vi "convert.vi"() -> ()   [LabVIEW 2013]
uses:
  errors/severity.ctl
  <vilib>/addons/JSON API/Variant JSON/Variant to JSON.vi
  <vilib>/addons/JSON API/JSON Value/Get as JSON string (pretty).vi
  errors/exception.lvlib
  <vilib>/addons/JSON API/Get Polymorphic/JSON GetSet.lvlib
  <vilib>/addons/JSON API/Variant JSON/Variant JSON.lvlib
  <vilib>/addons/JSON API/JSON Value/JSON Value.lvclass
panel:
  out "LabVIEW Text":string
  out "error in":errorcluster
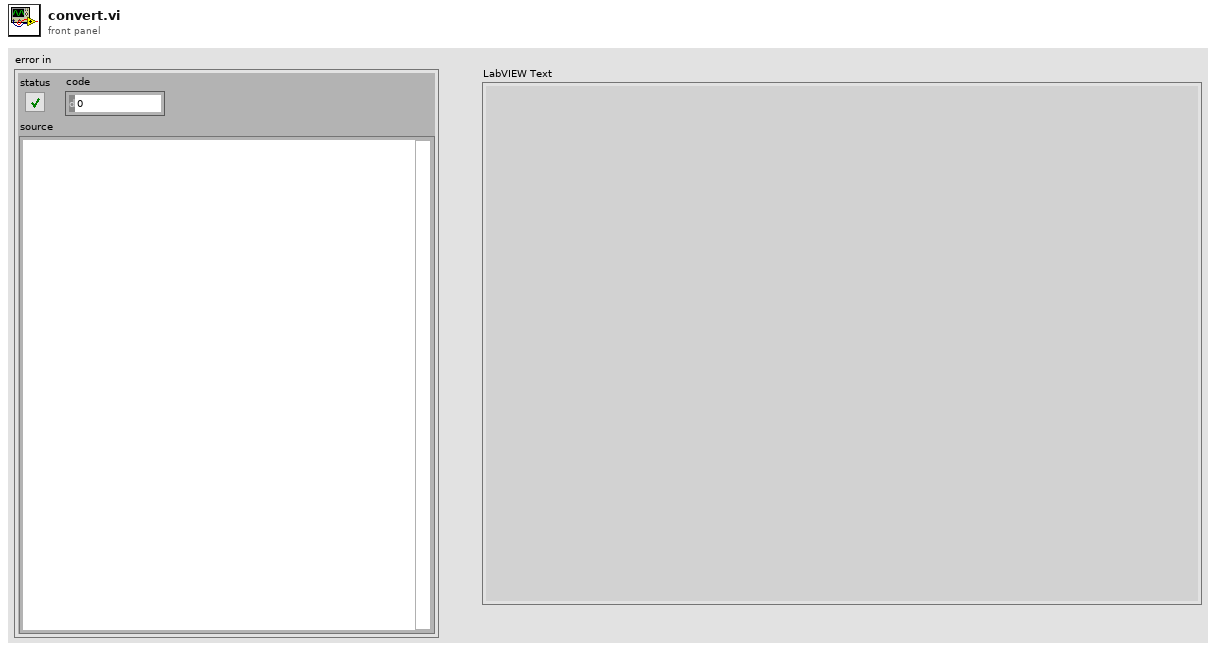
[diagram p1: front panel]
types:
  T1 = typedef "exception.lvlib/severity.ctl" = enum8{"unspecified", "operation failed", "data corruption", "system corruption", "critical unknown state"}
  T2 = typedef "exception.lvlib/exception.ctl" = cluster{"code":i32, "context":T3, "properties":variant}
  T3 = typedef "exception.lvlib/context.ctl" = enum16{"developer", "user interface", "standard", "limited", "deterministic"}
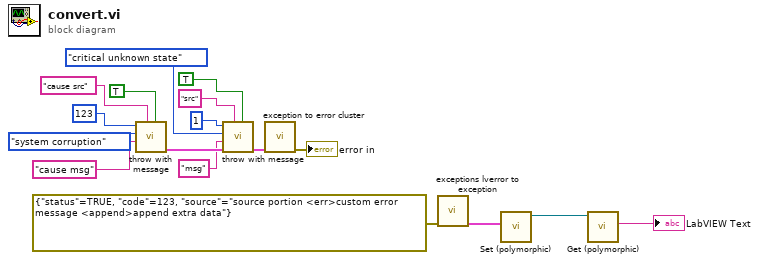
[diagram p0: block diagram]
diagram:
  n1 = call "throw with message.vi"("call chain?"=TRUE, "source"="cause src", "message"="cause msg", "severity"=severity."system corruption", "code"=123) -> ("exception out"=w9:T2)  [unwired: 6 in]
  n2 = call "throw with message.vi"("call chain?"=TRUE, "source"="src", "exception in"=w9, "message"="msg", "severity"=severity."critical unknown state", "code"=1) -> ("exception out"=w8:T2)  [unwired: 5 in]
  n3 = call "exception to error cluster.vi"("exception"=w8) -> ("error in"=→"error in":errorcluster)  [unwired: 10 in]
  n4 = call "exceptions lverror to exception.vi"("error in"=errorcluster {"status"=TRUE, "code"=123, "source"="source portion <err>custom error message <append>append extra data"}) -> ("exception"=w4:T2)  [unwired: 10 in]
  n5 = call-poly <vilib>:"Set (polymorphic).vi"("Variant"=w4) -> ("JSON Value out"=w6:refnum<class "JSON Value.lvclass">)  [unwired: 9 in, 1 out]
  n6 = call-poly <vilib>:"Get (polymorphic).vi"("JSON Value in"=w6) -> ("String"=→"LabVIEW Text":string)  [unwired: 9 in, 1 out]
